vi "FP_Get Monitor Indexes.vi"(8 "Primary":T2, 11 "All Work Spaces":T1=[{"Bounds"={"Left"=-10, "Top"=0, "Right"=0, "Bottom"=-10}, "Depth"=0}, {"Bounds"={"Left"=0, "Top"=0, "Right"=10, "Bottom"=10}, "Depth"=0}, {"Bounds"={"Left"=-10, "Top"=-10, "Right"=0, "Bottom"=0}, "Depth"=0}, {"Bounds"={"Left"=0, "Top"=-10, "Right"=10, "Bottom"=0}, "Depth"=0}, {"Bounds"={"Left"=10, "Top"=-10, "Right"=20, "Bottom"=0}, "Depth"=0}, {"Bounds"={"Left"=10, "Top"=0, "Right"=20, "Bottom"=10}, "Depth"=0}, {"Bounds"={"Left"=-10, "Top"=10, "Right"=0, "Bottom"=20}, "Depth"=0}, {"Bounds"={"Left"=0, "Top"=10, "Right"=10, "Bottom"=20}, "Depth"=0}, {"Bounds"={"Left"=10, "Top"=10, "Right"=20, "Bottom"=20}, "Depth"=0}]) -> (0 "Indexes Below Out":i32[](array[numeric]), 1 "Indexes Above Out":i32[](array[numeric]), 2 "Indexes Left Out":i32[](array[numeric]), 3 "Indexes Right Out":i32[](array[numeric]), 5 "Primary Index Out":i32)   [LabVIEW 2020]
uses:
  <vilib>/Utility/miscctls.llb/LVRectTypeDef.ctl
  <vilib>/Utility/miscctls.llb/LVAllMonitorsDisplayTypeDef.ctl
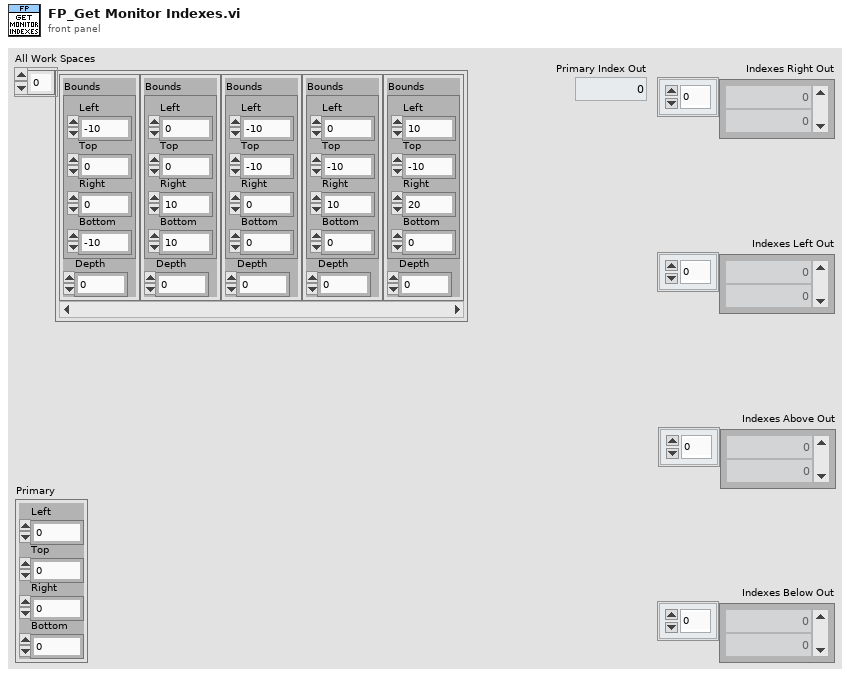
[diagram p1: front panel]
types:
  T1 = typedef "LVAllMonitorsDisplayTypeDef.ctl" = cluster{"Bounds":cluster{"Left":i16, "Top":i16, "Right":i16, "Bottom":i16}, "Depth":i16}[]
  T2 = typedef "LVRectTypeDef.ctl" = cluster{"Left":i16, "Top":i16, "Right":i16, "Bottom":i16}
  T3 = cluster{"Left":i16, "Top":i16, "Right":i16, "Bottom":i16}
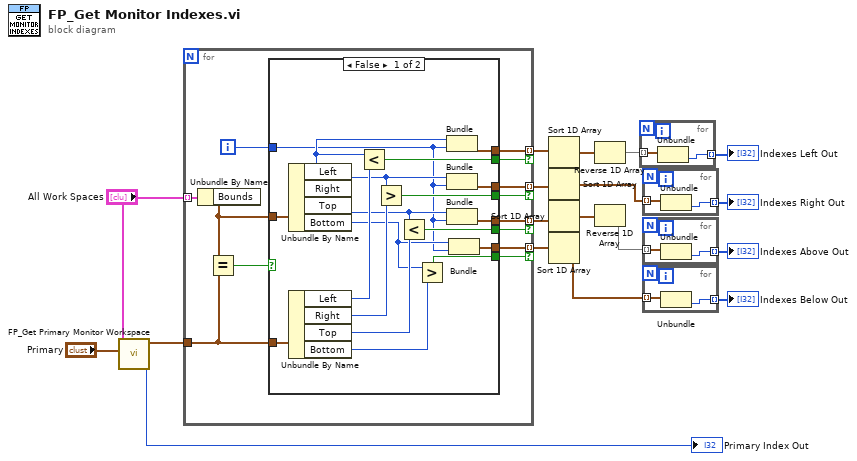
[diagram p0: block diagram]
diagram:
  n1 = call "FP_Get Primary Monitor Workspace.vi"("Primary"="Primary", "All Work Spaces"="All Work Spaces") -> ("Index Out"=→"Primary Index Out":i32, "Primary Work Space Out"=w2:T3)  [unwired: 8 in]
  n2 = for {
    tunnel: "All Work Spaces" -> [w31] mode=indexing
    tunnel: w2 -> [w20]
    tunnel: [w26] -> w18 mode=indexing if=w29
    tunnel: [w24] -> w16 mode=indexing if=w28
    tunnel: [w23] -> w15 mode=indexing if=w27
    tunnel: [w22] -> w14 mode=indexing if=w25
    i -> [w30]
    n3 = Unbundle By Name(w31) -> ("Bounds"=w21:T3)
    n4 = Equal?(x=w21, y=w20) -> (x = y?=w19:bool)
    n5 = case shown="False" w19 {
      tunnel: w21 -> [w50 _]
      tunnel: w20 -> [w49 _]
      tunnel: w30 -> [w33 _]
      tunnel: [w39 _] -> w26
      tunnel: [w47 _] -> w29
      tunnel: [w45 _] -> w28
      tunnel: [w43 _] -> w27
      tunnel: [w41 _] -> w25
      tunnel: [w37 _] -> w24
      tunnel: [w35 _] -> w23
      tunnel: [w32 _] -> w22
      frame False {
        n6 = Unbundle By Name(w50) -> ("Left"=w40:i16, "Right"=w38:i16, "Top"=w36:i16, "Bottom"=w34:i16)
        n7 = Unbundle By Name(w49) -> ("Left"=w48:i16, "Right"=w46:i16, "Top"=w44:i16, "Bottom"=w42:i16)
        n8 = Less?(x=w40, y=w48) -> (x < y?=w47:bool)
        n9 = Greater?(x=w38, y=w46) -> (0:w45:bool)
        n10 = Less?(x=w36, y=w44) -> (x < y?=w43:bool)
        n11 = Greater?(x=w34, y=w42) -> (0:w41:bool)
        n12 = Bundle("Left"=w40, w33) -> (w39:cluster{"Left":i16, i32})  [unwired: 1 in]
        n13 = Bundle("Right"=w38, w33) -> (w37:cluster{"Right":i16, i32})  [unwired: 1 in]
        n14 = Bundle("Top"=w36, w33) -> (w35:cluster{"Top":i16, i32})  [unwired: 1 in]
        n15 = Bundle("Bottom"=w34, w33) -> (w32:cluster{"Bottom":i16, i32})  [unwired: 1 in]
      }
      frame True {
      }
    }
  }
  n16 = Sort 1D Array(array=w18) -> (sorted array=w17:cluster{"Left":i16, i32}[])
  n17 = Sort 1D Array(array=w16) -> (sorted array=w10:cluster{"Right":i16, i32}[])
  n18 = Sort 1D Array(array=w15) -> (sorted array=w13:cluster{"Top":i16, i32}[])
  n19 = Sort 1D Array(array=w14) -> (sorted array=w6:cluster{"Bottom":i16, i32}[])
  n20 = Reverse 1D Array(array=w17) -> (reversed array=w12:cluster{"Left":i16, i32}[])
  n21 = Reverse 1D Array(array=w13) -> (reversed array=w8:cluster{"Top":i16, i32}[])
  n22 = for {
    tunnel: w12 -> [w52] mode=indexing
    tunnel: [w51] -> w11 mode=indexing
    n23 = Unbundle(w52) -> (w51:i32)  [unwired: 1 out]
  }
  "Indexes Left Out" <- w11
  n24 = for {
    tunnel: w10 -> [w54] mode=indexing
    tunnel: [w53] -> w9 mode=indexing
    n25 = Unbundle(w54) -> (w53:i32)  [unwired: 1 out]
  }
  "Indexes Right Out" <- w9
  n26 = for {
    tunnel: w8 -> [w56] mode=indexing
    tunnel: [w55] -> w7 mode=indexing
    n27 = Unbundle(w56) -> (w55:i32)  [unwired: 1 out]
  }
  "Indexes Above Out" <- w7
  n28 = for {
    tunnel: w6 -> [w58] mode=indexing
    tunnel: [w57] -> w5 mode=indexing
    n29 = Unbundle(w58) -> (w57:i32)  [unwired: 1 out]
  }
  "Indexes Below Out" <- w5
